vi "Stop Threshold Actor.vi"(8 "error in (no error)":errorcluster, 11 "Threshold in":refnum<class "Threshold.lvclass">) -> (0 "error out":errorcluster, 3 "Threshold out":refnum<class "Threshold.lvclass">)   [LabVIEW 2016, in "Tests.lvlib" / "Threshold.lvclass"]
uses:
  Threshold.lvclass
  Threshold.lvclass/Threshold.ctl
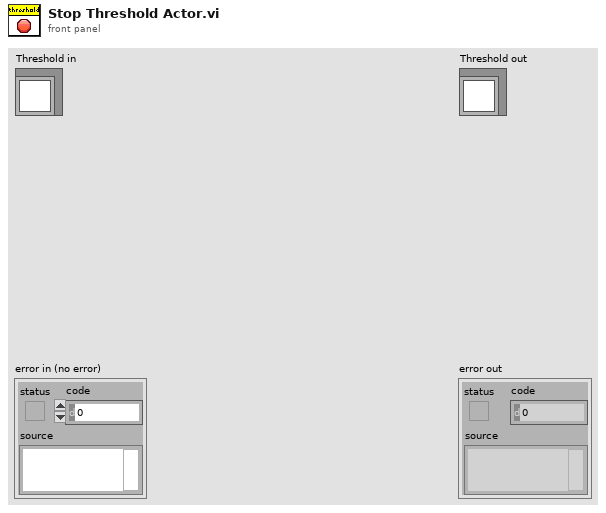
[diagram p1: front panel]
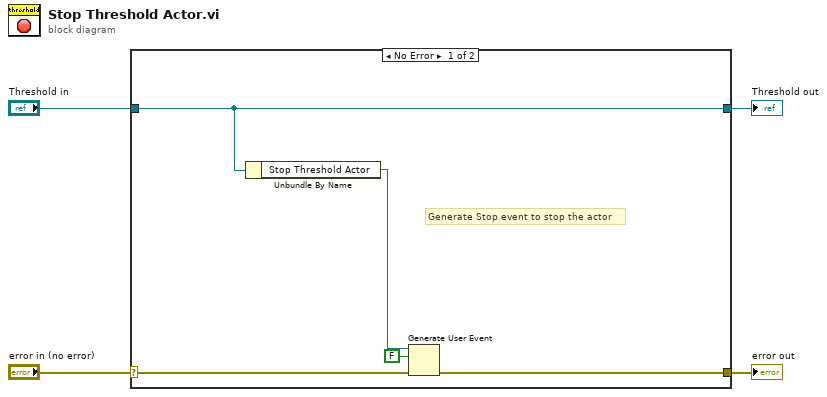
[diagram p0: block diagram]
diagram:
  n1 = case shown="No Error" "error in (no error)" {
    selector: "error in (no error)" -> [w8 w11]
    tunnel: [w7 w11] -> w3
    tunnel: [w9 w10] -> w1
    tunnel: "Threshold in" -> [w9 w10]
    frame No Error {
      # "Generate Stop event to stop the actor"
      n2 = Unbundle By Name(w9) -> ("Stop Threshold Actor"=w6:refnum<user-event>)
      n3 = Generate User Event(user event=w6, event data cluster=FALSE ("event data"), error in=w8) -> (error out=w7:errorcluster)  [unwired: 1 in, 1 out]
    }
    frame Error {
    }
  }
  "error out" <- w3
  "Threshold out" <- w1
